vi "Validate Instrument Revision.vi"(0 "VISA resource name":refnum<visa-resource-name>, 11 "error in (no error)":errorcluster) -> (4 "VISA resource name out":refnum<visa-resource-name>, 6 "Firmware Version":string, 10 "Model Number":T1(ring), 15 "error out":errorcluster)   [LabVIEW 2014, in "Associated Power Technologies 8500 Series.lvlib"]
doc: "Queries the instrument for the model number and firmware revision and validates them."
uses:
  <instrlib>/Associated Power Technologies 8500 Series/Associated Power Technologies 8500 Series.lvlib
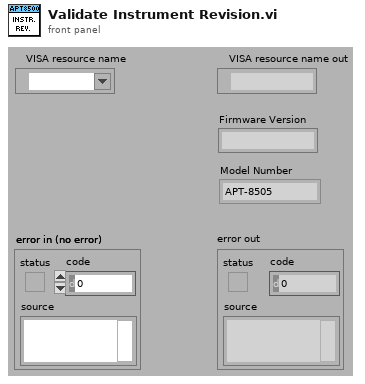
[diagram p1: front panel]
types:
  T1 = enum16{"APT-8505", "APT-8512", "APT-8520", "APT-8540"}
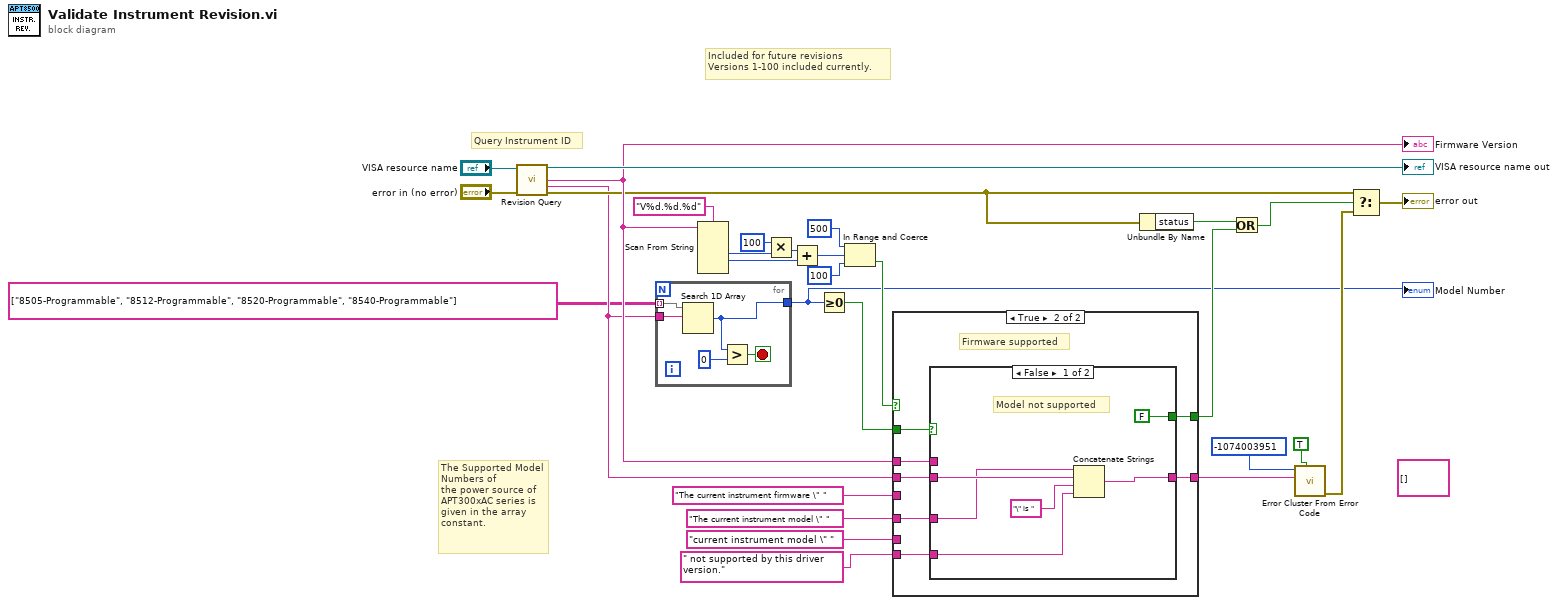
[diagram p0: block diagram]
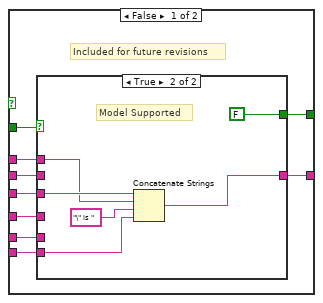
[diagram p2: hidden frame]
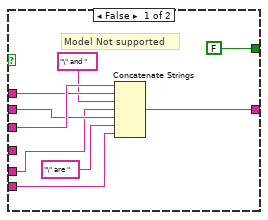
[diagram p3: hidden frame]
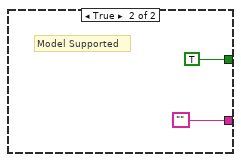
[diagram p4: hidden frame]
diagram:
  (unwired) string[][] []
  # "Included for future revisions\nVersions 1-100 included currently."
  # "The Supported Model Numbers of\nthe power source of APT300xAC series is given in the array constant."
  # "Query Instrument ID"
  n1 = call <instrlib>:"Revision Query.vi"("VISA resource name"="VISA resource name", "error in (no error)"="error in (no error)") -> ("VISA resource name out"=→"VISA resource name out":refnum<visa-resource-name>, "Instrument Firmware Revision"=w12:string, "Instrument Model"=w3:string, "error out"=w4:errorcluster)  [unwired: 9 in, 1 out]
  "Firmware Version" <- w12
  n2 = for {
    tunnel: [w32] -> w1
    tunnel: w3 -> [w35]
    tunnel: string[][] [["8505-Programmable", "8512-Programmable", "8520-Programmable", "8540-Programmable"]] -> [w34] mode=indexing
    stop <- w31 stop-if-true
    n3 = Search 1D Array(1D array=w34, element=w35) -> (index of element=w32:i32)  [unwired: 1 in]
    n4 = Greater?(x=w32, y=0) -> (0:w31:bool)
  }
  "Model Number" <- w1
  n5 = Scan From String(format string="V%d.%d.%d", input string=w12) -> (output 1=w11:i32, output 2=w8:i32)  [unwired: 6 in, 3 out]
  n6 = Multiply(x=100 ("y"), y=w11) -> (x*y=w9:i32)
  n7 = Add(x=w9, y=w8) -> (x+y=w7:i32)
  n8 = Greater Or Equal To 0?(x=w1) -> (x >= 0?=w24:bool)
  n9 = In Range and Coerce(upper limit=500, x=w7, lower limit=100) -> (In Range?=w15:bool)  [unwired: 1 out]
  n10 = case shown="True" w15 {
    tunnel: w24 -> [w43 w66]
    tunnel: w3 -> [w44 w65]
    tunnel: w12 -> [w42 w64]
    tunnel: " not supported by this driver version." ("Source (VI Name)") -> [w41 w62]
    tunnel: "The current instrument model \" " ("Source (VI Name)") -> [w40 w63]
    tunnel: "The current instrument firmware \" " ("Source (VI Name)") -> [w39 _]
    tunnel: [w38 w61] -> w20
    tunnel: [w37 w60] -> w18
    tunnel: "current instrument model \" " ("Source (VI Name)") -> [w36 _]
    frame False {
      # "Included for future revisions"
      n11 = case shown="True" w43 {
        tunnel: w44 -> [w51 _]
        tunnel: w42 -> [w52 w58]
        tunnel: w41 -> [w50 w56]
        tunnel: w40 -> [_ _]
        tunnel: w39 -> [w53 w59]
        tunnel: [w47 w54] -> w38
        tunnel: [FALSE ("show call chain? (False)") FALSE ("show call chain? (False)")] -> w37
        tunnel: w36 -> [w45 _]
        frame False {
          # "Model Not supported"
          n12 = Concatenate Strings(w53, w52, "\" and " ("string"), w45, w51, "\" are " ("Source (VI Name)"), w50) -> (w47:string)
        }
        frame True {
          # "Model Supported"
          n13 = Concatenate Strings(w59, w58, "\" is " ("string"), w56) -> (w54:string)
        }
      }
    }
    frame True {
      # "Firmware supported"
      n14 = case shown="False" w66 {
        tunnel: w65 -> [w71 _]
        tunnel: w64 -> [_ _]
        tunnel: w63 -> [w70 _]
        tunnel: w62 -> [w69 _]
        tunnel: [w68 ""] -> w61
        tunnel: [FALSE TRUE] -> w60
        frame False {
          # "Model not supported"
          n15 = Concatenate Strings(w70, w71, "\" is " ("string"), w69) -> (w68:string)
        }
        frame True {
          # "Model Supported"
        }
      }
    }
  }
  n16 = Unbundle By Name(w4) -> ("status"=w17:bool)
  n17 = Or(x=w17, y=w18) -> (x .or. y?=w16:bool)
  n18 = call <vilib>:"Error Cluster From Error Code.vi"("show call chain? (False)"=TRUE, "error message (\"\")"=w20, "error code (0)"=-1074003951 ("Code")) -> ("error out"=w28:errorcluster)  [unwired: 6 in]
  n19 = Select(t=w4, s=w16, f=w28) -> (s? t:f=→"error out":errorcluster)
